vi "Write DMA.vi"(1 "FIFO In":refnum<k21>="T2H", 5 "16xU32":u32[](array[numeric])=[0, 0, 0, 0, 0, 0, 0, 0, 0, 0, 0, 0, 0, 0, 0, 0], 9 "input valid":bool) -> (10 "Timed Out?":bool)   [LabVIEW 2015, in "DDC_7976R_v1.lvlib"]
doc: "This VI is waiting for 16 valid samples, one-by-one.\nWhen 16 samples have arrived then it writes them into DMA FIFO."
uses:
  DDC_7976R_v1.lvlib
  <vilib>/rvi/DataTransferAndStorage/Container/Common/niFpgaContainerExecOnDevCompGetState.vi
  <vilib>/rvi/Emulation/niFpgaSctlEmulationGetInTimedLoop.vi
  <vilib>/rvi/errors/niFpgaSetErrorForExecOnDevCompSimple.vi
  <vilib>/rvi/eio/common/nirviEmuReportErrorAndStop.vi
  <vilib>/rvi/interface/RandomDataEmulation/nirviRandomDataAcquireLock.vi
  <vilib>/rvi/interface/RandomDataEmulation/nirviRandomDataQueueStore.vi
  <vilib>/rvi/interface/RandomDataEmulation/nirviRandomDataReleaseLock.vi
  <vilib>/rvi/interface/RandomDataEmulation/nirviFPGAContextMergeError.vi
  <vilib>/rvi/interface/RandomDataEmulation/nirviRandomDataCheckExitLoopConditions.vi
  <vilib>/express/rvi/timingcommon/nirviCommon.vi
  <vilib>/rvi/interface/RandomDataEmulation/niFpgaRandomDataHandleErrors.vi
  <vilib>/rvi/DataTransferAndStorage/Container/XNode/niFpgaContainer.xnode
  <vilib>/rvi/FIFO/Fifo_Resource/niFpgaFifoEmulationRefInMultiElement.vi
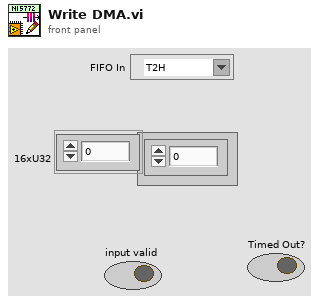
[diagram p1: front panel]
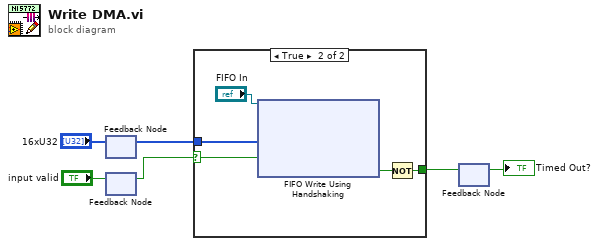
[diagram p0: block diagram]
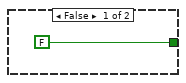
[diagram p2: hidden frame]
diagram:
  n1 = feedback #1() -> (w3:u32[])  [unwired: 1 in]
  n2 = feedback-in #1("16xU32") -> ()
  n3 = feedback #2() -> (w5:bool)  [unwired: 1 in]
  n4 = feedback-in #2("input valid") -> ()
  n5 = case shown="True" w5 {
    selector: w5 -> [_ w8]
    tunnel: [FALSE ("Timed Out?") w12] -> w2
    tunnel: w3 -> [_ w9]
    frame False {
    }
    frame True {
      n6 = xnode ("FIFO Write Using Handshaking")("Element"=w9, "Input Valid"=w8, "FIFO In"="FIFO In") -> ("Ready for Input"=w10:bool)  [unwired: 1 out]
      n7 = Not(x=w10) -> (.not. x?=w12:bool)
    }
  }
  n8 = feedback-in #3(w2) -> ()
  n9 = feedback #3() -> (→"Timed Out?":bool)  [unwired: 1 in]
